vi "Double to String.vi"(10 "Double In":dbl=0.0002 format="%#_13g") -> (2 "String Value":string)   [LabVIEW 2023, in "NI PXIe-411x PS Custom Device.lvlib"]
uses:
  NI PXIe-411x PS Custom Device.lvlib
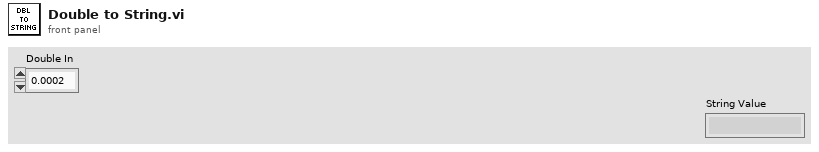
[diagram p1: front panel]
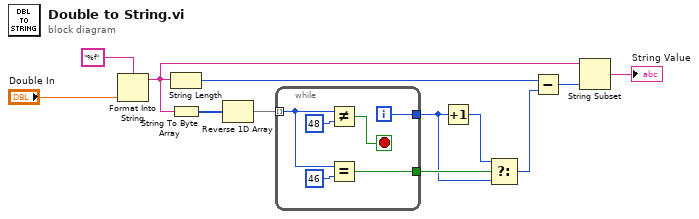
[diagram p0: block diagram]
diagram:
  n1 = Format Into String(format string="%f", "Double In") -> (resulting string=w7:string)  [unwired: 2 in, 1 out]
  n2 = String Length(string=w7) -> (length=w8:i32)
  n3 = String To Byte Array(string=w7) -> (unsigned byte array=w10:u8[])
  n4 = Reverse 1D Array(array=w10) -> (reversed array=w9:u8[])
  n5 = while {
    tunnel: w9 -> [w15] mode=indexing
    tunnel: [w16] -> w3
    tunnel: [w13] -> w4
    i -> [w16]
    stop <- w17 stop-if-true
    n6 = Not Equal?(x=w15, y=u8 48) -> (x != y?=w17:bool)
    n7 = Equal?(x=w15, y=u8 46) -> (x = y?=w13:bool)
  }
  n8 = Increment(x=w3) -> (x+1=w2:i32)
  n9 = Select(t=w2, s=w4, f=w3) -> (s? t:f=w1:i32)
  n10 = Subtract(x=w8, y=w1) -> (x-y=w6:i32)
  n11 = String Subset(string=w7, length (rest)=w6) -> (substring=→"String Value":string)  [unwired: 1 in]
